vi "SalcompMESCheck Process.vi"(5 "SN":string, 11 "错误输入（无错误）":errorcluster) -> (6 "Message":string, 10 "CheckRouteForSerialNumber":bool, 15 "错误输出":errorcluster)   [LabVIEW 2018]
uses:
  CMESAPI.dll
panel:
  # "C:\\Users\\cnastest1\\AppData\\Local\\assembly\\dl3\\2HZ36AHX.O4G\\7ABBNLA9.Y2Y\\af183ff5\\00f4eecf_d193d601"
  # "KF5512M4V99999"
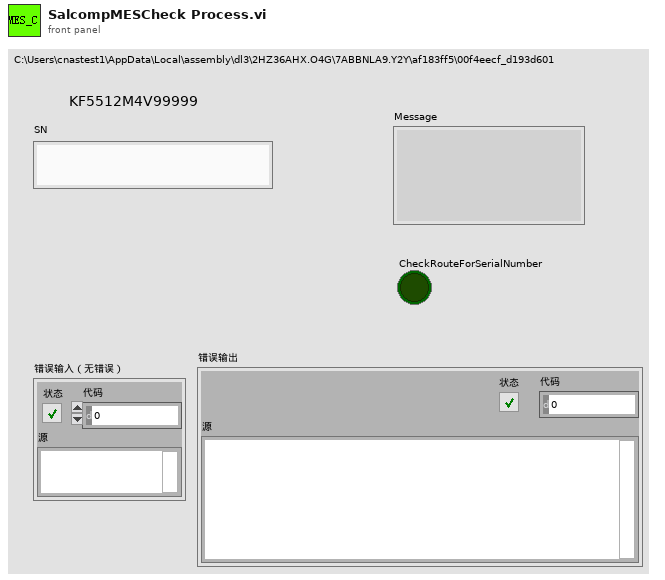
[diagram p1: front panel]
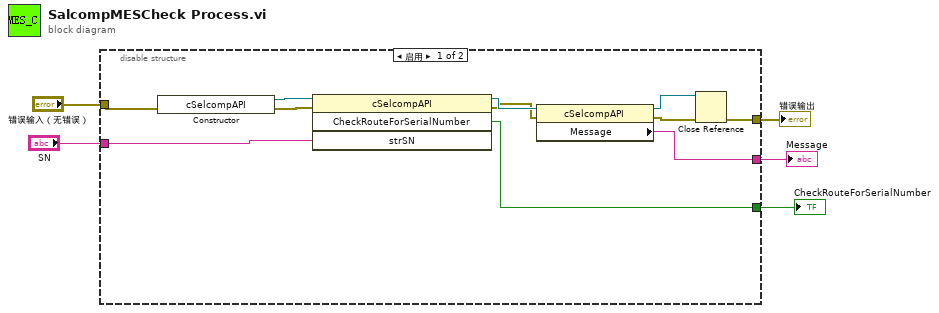
[diagram p0: block diagram]
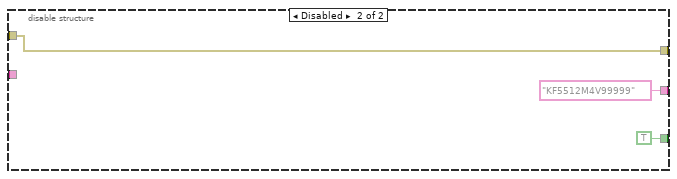
[diagram p2: hidden frame]
diagram:
  n1 = disable-structure shown="启用" {
    disable-tunnel: "SN" -> [w10 _]
    disable-tunnel: [w9 TRUE ("CheckRouteForSerialNumber")] -> w4
    disable-tunnel: [w8 "KF5512M4V99999" ("Message")] -> w3
    disable-tunnel: "错误输入（无错误）" -> [w7 w17]
    disable-tunnel: [w6 w17] -> w1
    frame Enabled {
      n2 = constructor class="cSelcompAPI"(error in=w7) -> (reference out=w16:refnum<k24>, error out=w15:errorcluster)  [unwired: 2 in, 1 out]
      n3 = invoke class="cSelcompAPI" method="CheckRouteForSerialNumber"(reference=w16, error in=w15, "strSN"=w10) -> (reference out=w14:refnum<k24>, error out=w13:errorcluster, "CheckRouteForSerialNumber"=w9:bool)  [unwired: 1 in, 1 out]
      n4 = property class="cSelcompAPI"(reference=w14, error in=w13) -> (reference out=w12:refnum<k24>, error out=w11:errorcluster, "Message"=w8:string)
      n5 = Close Reference(reference=w12, error in (no error)=w11) -> (error out=w6:errorcluster)
    }
    frame Disabled {
    }
  }
  "CheckRouteForSerialNumber" <- w4
  "Message" <- w3
  "错误输出" <- w1
